vi "Within Limits.vi"(9 "Input":dbl, 10 "Bottom Switch":bool, 11 "Top Switch":bool) -> (3 "Output":dbl)   [LabVIEW 2014]
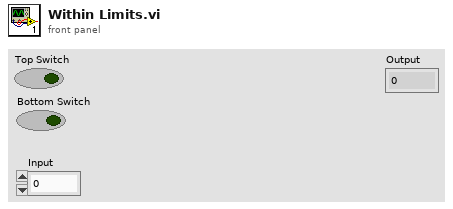
[diagram p1: front panel]
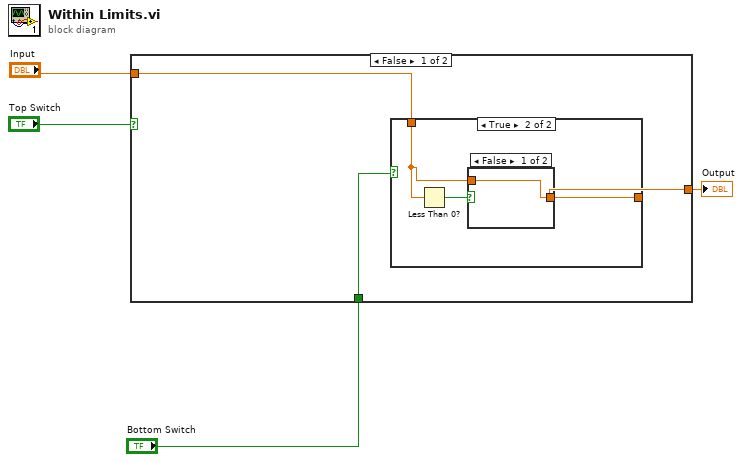
[diagram p0: block diagram]
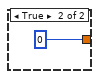
[diagram p3: hidden frame]
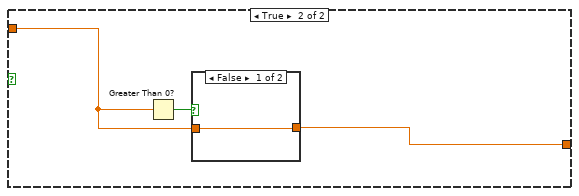
[diagram p4: hidden frame]
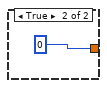
[diagram p5: hidden frame]
diagram:
  n1 = case shown="False" "Top Switch" {
    tunnel: "Input" -> [w7 w14]
    tunnel: [w6 w15] -> w2
    tunnel: "Bottom Switch" -> [w5 _]
    frame False {
      n2 = case shown="True" w5 {
        tunnel: w7 -> [w8 w9]
        tunnel: [w8 w10] -> w6
        frame False {
        }
        frame True {
          n3 = Less Than 0?(x=w9) -> (x < 0?=w11:bool)
          n4 = case shown="False" w11 {
            tunnel: [w12 0] -> w10
            tunnel: w9 -> [w12 _]
            frame False {
            }
            frame True {
            }
          }
        }
      }
    }
    frame True {
      n5 = Greater Than 0?(x=w14) -> (x > 0?=w16:bool)
      n6 = case shown="False" w16 {
        tunnel: [w17 0] -> w15
        tunnel: w14 -> [w17 _]
        frame False {
        }
        frame True {
        }
      }
    }
  }
  "Output" <- w2
